vi "Agilent U2722 - TEST 3 Channel Output.vi"() -> ()   [LabVIEW 2010]
doc: "This example shows how to configure the instrument's output voltage level, over current protection, and over voltage protection. The actual voltage level and actual current level are returned as well as whether over voltage protection (OVP) or over current protection (OCP) has been tripped."
uses:
  Agilent U2722.lvlib
panel:
  out "Actual Voltage":dbl format="%0.2f"
  out "error out":errorcluster
  out "Update Time":u32
  in  "Output Level (1.0 mA)":dbl
  out "Actual Current (mA)":dbl format="%.2f"
  in  "VISA resource name":refnum<visa-resource-name>="Agilent"
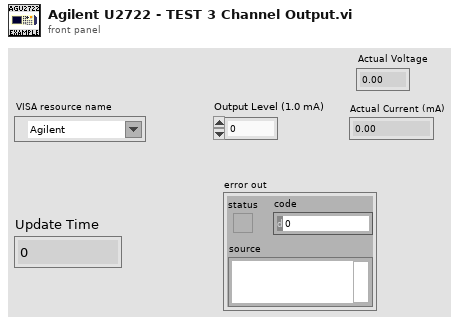
[diagram p1: front panel]
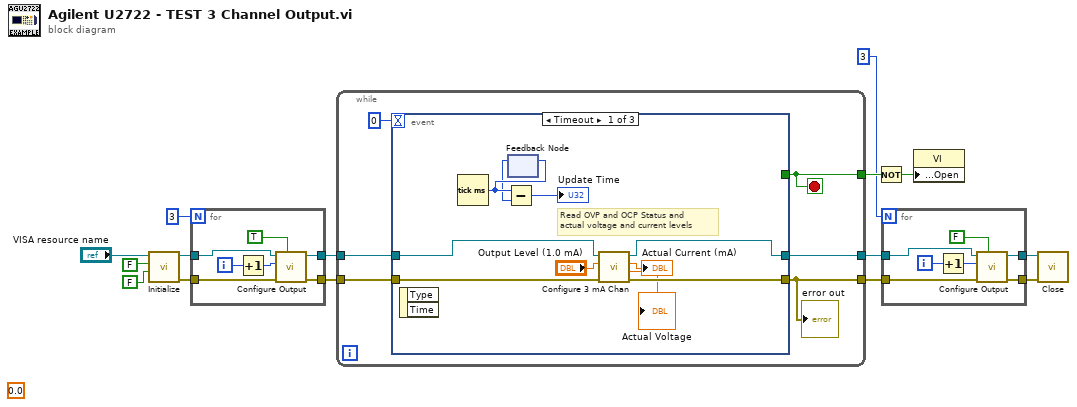
[diagram p0: block diagram]
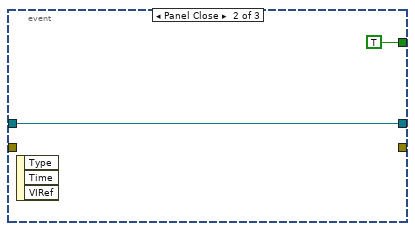
[diagram p2: hidden frame]
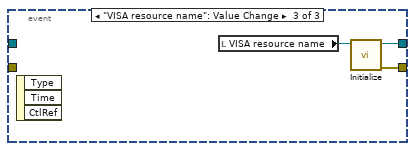
[diagram p3: hidden frame]
diagram:
  (unwired) 0.0
  n1 = call "Initialize.vi"("Reset (True)"=FALSE, "ID Query (True)"=FALSE, "VISA resource name"="VISA resource name") -> ("error out"=w9:errorcluster, "VISA resource name out"=w10:refnum<visa-resource-name>)  [unwired: 7 in]
  n2 = for {
    N: 3 -> [_]
    tunnel: w10 -> [w22]
    tunnel: w9 -> [w21]
    tunnel: [w20] -> w8
    tunnel: [w19] -> w7
    i -> [w18]
    n3 = Increment(x=w18) -> (x+1=w17:i32)
    n4 = call "Configure Output.vi"("Enable Output (T: Enable)"=TRUE, "error in (no error)"=w21, "Channel (1: Channel 1)"=w17, "VISA resource name"=w22) -> ("error out"=w19:errorcluster, "VISA resource name out"=w20:refnum<visa-resource-name>)  [unwired: 6 in]
  }
  n5 = while {
    tunnel: w8 -> [w26]
    tunnel: w7 -> [w25]
    tunnel: [w28] -> w2
    tunnel: [w27] -> w1
    tunnel: [w24] -> w12
    stop <- w24 stop-if-true
    n6 = event shown="[0] Timeout" {
      selector: _ -> [_ _ _]
      dyn-events: _ -> [_ _ _]
      timeout: 0 -> [_ _ _]
      tunnel: [w38 w39 w41] -> w28
      tunnel: [w30 _ w42] -> w27
      tunnel: w26 -> [w37 w39 _]
      tunnel: w25 -> [w36 _ _]
      tunnel: [_ TRUE ("status") _] -> w24
      event Timeout {
        # "Read OVP and OCP Status and\nactual voltage and current levels"
        n7 = event-data() -> ()  [unwired: 1 in, 2 out]
        n8 = Tick Count (ms)() -> (millisecond timer value=w33:u32)
        n9 = feedback-in #1(w33) -> ()
        n10 = feedback #1() -> (w32:u32)  [unwired: 1 in]
        n11 = Subtract(x=w33, y=w32) -> (x-y=→"Update Time":u32)
        n12 = call "Configure 3 mA Chan.vi"("error In"=w36, "Output Level (1.0 mA)"="Output Level (1.0 mA)", "VISA resource name in"=w37) -> ("error out"=w30:errorcluster, "Voltage"=→"Actual Voltage":dbl, "Actual mA Out"=→"Actual Current (mA)":dbl, "VISA resource name out"=w38:refnum<visa-resource-name>)  [unwired: 5 in]
      }
      event Panel Close {
        n13 = event-data() -> ()  [unwired: 1 in, 3 out]
      }
      event "VISA resource name": Value Change {
        n14 = event-data() -> ()  [unwired: 1 in, 3 out]
        n15 = local read "VISA resource name"() -> (w43:refnum<visa-resource-name>)
        n16 = call "Initialize.vi"("VISA resource name"=w43) -> ("error out"=w42:errorcluster, "VISA resource name out"=w41:refnum<visa-resource-name>)  [unwired: 9 in]
      }
    }
    "error out" <- w27
  }
  n17 = Not(x=w12) -> (.not. x?=w11:bool)
  n18 = for {
    N: 3 -> [_]
    tunnel: w2 -> [w50]
    tunnel: w1 -> [w49]
    tunnel: [w48] -> w4
    tunnel: [w47] -> w3
    i -> [w46]
    n19 = Increment(x=w46) -> (x+1=w45:i32)
    n20 = call "Configure Output.vi"("Enable Output (T: Enable)"=FALSE, "error in (no error)"=w49, "Channel (1: Channel 1)"=w45, "VISA resource name"=w50) -> ("error out"=w47:errorcluster, "VISA resource name out"=w48:refnum<visa-resource-name>)  [unwired: 6 in]
  }
  n21 = property class="VI"("Front Panel.Open"=w11) -> ()  [unwired: 2 in, 2 out]
  n22 = call "Close.vi"("error in (no error)"=w3, "VISA resource name"=w4) -> ()  [unwired: 9 in, 1 out]
